vi "DB Tools Get Types From File.vi"(4 "error in (no error)":errorcluster) -> (0 "error out":errorcluster, 3 "data types":string[](array[string]))   [LabVIEW 2012, in "NI_Database_API_64.lvlib"]
doc: "Returns the data types (array of strings) listed in the dbtypes.ini file located in the LabVIEW\\database directory."
uses:
  NI_Database_API_64.lvlib
  DB Tools SQL Server Types.ctl
  DB Tools DataTypes.ctl
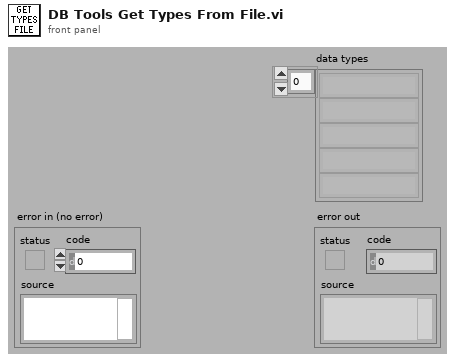
[diagram p1: front panel]
types:
  T1 = enum16{"read/write", "read-only", "write-only", "write-only (truncate)"}
  T2 = typedef "NI_Database_API_64.lvlib/DB Tools SQL Server Types.ctl" = enum16{"varchar", "integer", "real", "float", "datetime", "image"}
  T3 = typedef "NI_Database_API_64.lvlib/DB Tools DataTypes.ctl" = enum16{"String", "Long (I32)", "Single (SGL)", "Double (DBL)", "Date/Time", "Binary"}
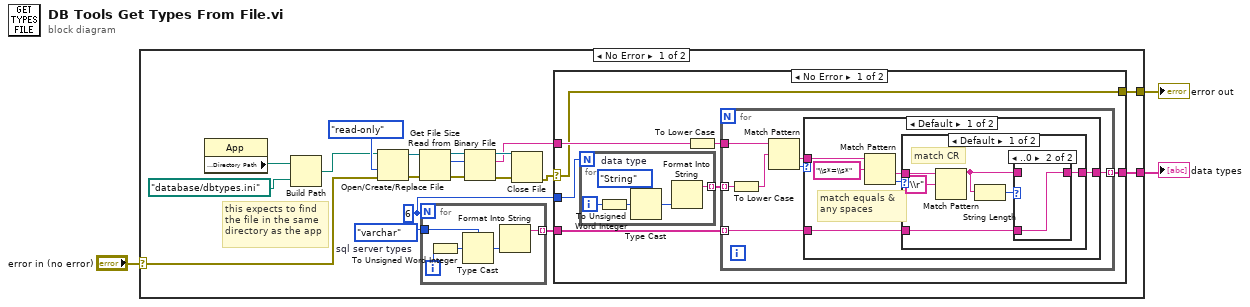
[diagram p0: block diagram]
diagram:
  n1 = case shown="No Error" "error in (no error)" {
    selector: "error in (no error)" -> [w5 w65]
    tunnel: [w17 w65] -> w3
    tunnel: [w6 _] -> w2
    frame No Error {
      w9 = DB_Tools_SQL_Server_Types."varchar"  # sql server types
      w7 = 6
      # "this expects to find \nthe file in the same \ndirectory as the app"
      n2 = property class="App"() -> ("Application:Directory Path"=w12:path)  [unwired: 2 in, 2 out]
      n3 = Build Path(base path=w12, name or relative path=path "database/dbtypes.ini" ("Path")) -> (appended path=w10:path)
      n4 = Open/Create/Replace File(file path (use dialog)=w10, error in=w5, access (0:read/write)=T1."read-only" ("open mode (0)")) -> (refnum out=w15:refnum<file>, error out=w13:errorcluster)  [unwired: 3 in, 1 out]
      n5 = Get File Size(file=w15, error in=w13) -> (refnum out=w16:refnum<file>, size (in bytes)=w4:i64, 0:w14:errorcluster)
      n6 = for {
        N: w7 -> [_]
        tunnel: [w24] -> w8 mode=indexing
        tunnel: w9 -> [w23]
        i -> [w27]
        n7 = To Unsigned Word Integer(number=w27) -> (unsigned 16bit integer=w26:u16)
        n8 = Type Cast(type=w23, x=w26) -> (*(type *) &x=w25:T2)
        n9 = Format Into String(w25) -> (resulting string=w24:string)  [unwired: 3 in, 1 out]
      }
      n10 = Read from Binary File(8:w14, 10:w4, 11:w16) -> (0:w22:errorcluster, 2:w19:string, 3:w21:refnum<file>)  [unwired: 3 in, 1 out]
      n11 = Close File(refnum=w21, error in=w22) -> (error out=w18:errorcluster)  [unwired: 1 out]
      n12 = case shown="No Error" w18 {
        selector: w18 -> [w30 w63]
        tunnel: w19 -> [w33 _]
        tunnel: [w32 w64] -> w6
        tunnel: w8 -> [w31 w64]
        tunnel: [w30 w63] -> w17
        tunnel: w7 -> [w28 _]
        frame No Error {
          n13 = for {
            N: w28 -> [_]
            tunnel: [w36] -> w29 mode=indexing
            i -> [w39]
            w35 = DB_Tools_DataTypes."String"  # data type
            n14 = To Unsigned Word Integer(number=w39) -> (unsigned 16bit integer=w38:u16)
            n15 = Type Cast(type=w35, x=w38) -> (*(type *) &x=w37:T3)
            n16 = Format Into String(w37) -> (resulting string=w36:string)  [unwired: 3 in, 1 out]
          }
          n17 = To Lower Case(string=w33) -> (all lower case string=w34:string)
          n18 = for {
            tunnel: w29 -> [w42] mode=indexing
            tunnel: w34 -> [w46]
            tunnel: [w43] -> w32 mode=indexing
            tunnel: w31 -> [w40] mode=indexing
            n19 = To Lower Case(string=w42) -> (all lower case string=w41:string)
            n20 = Match Pattern(string=w46, regular expression=w41) -> (after substring=w44:string, offset past match=w45:i32)  [unwired: 1 in, 2 out]
            n21 = case shown="Default" w45 {
              tunnel: w44 -> [w52 _]
              tunnel: [w48 w62] -> w43
              tunnel: w40 -> [w47 w62]
              frame Default {
                # "match equals & \nany spaces"
                n22 = Match Pattern(string=w52, regular expression="\\s*=\\s*") -> (after substring=w49:string, offset past match=w50:i32)  [unwired: 1 in, 2 out]
                n23 = case shown="Default" w50 {
                  tunnel: w49 -> [w58 _]
                  tunnel: [w55 w61] -> w48
                  tunnel: w47 -> [w53 w61]
                  frame Default {
                    # "match CR"
                    n24 = Match Pattern(string=w58, regular expression="\\r") -> (before substring=w54:string)  [unwired: 1 in, 3 out]
                    n25 = String Length(string=w54) -> (length=w56:i32)
                    n26 = case shown="..0" w56 {
                      tunnel: [w59 w60] -> w55
                      tunnel: w54 -> [w59 _]
                      tunnel: w53 -> [_ w60]
                      frame Default {
                      }
                      frame ..0 {
                      }
                    }
                  }
                  frame -1 {
                    # "not found"
                  }
                }
              }
              frame -1 {
                # "not found"
              }
            }
          }
        }
        frame Error {
        }
      }
    }
    frame Error {
    }
  }
  "error out" <- w3
  "data types" <- w2
